vi "Log.StorePaths.vi"(8 "error in (no error)":errorcluster, 10 "TestStand Version (2013)":string, 11 "VeriStand Version (2013 SP1)":string) -> (0 "error out":errorcluster)   [LabVIEW 2013]
uses:
  <vilib>/Utility/sysdir.llb/System Directory Type.ctl
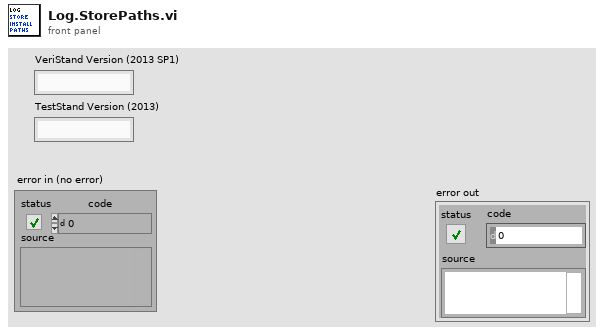
[diagram p1: front panel]
types:
  T1 = typedef "System Directory Type.ctl" = i32
  T2 = enum16{"open", "replace", "create", "open or create", "replace or create", "replace or create with confirmation"}
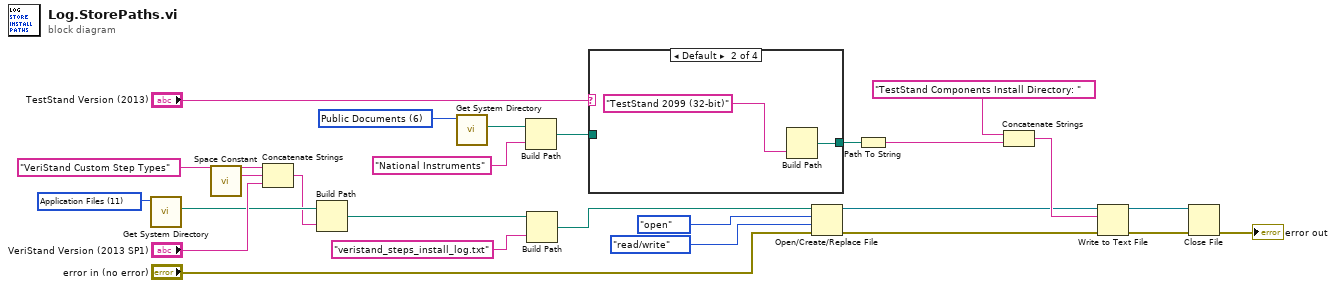
[diagram p0: block diagram]
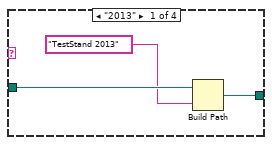
[diagram p2: hidden frame]
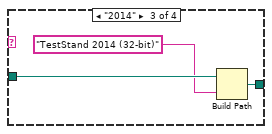
[diagram p3: hidden frame]
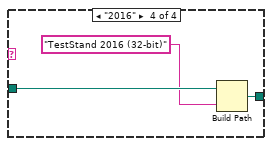
[diagram p4: hidden frame]
diagram:
  w18 = T1 6 items=["User Home"=0, "User Desktop"=1, "User Documents"=2, "User Application Data"=3, "User Preferences"=4, "User Temporary"=5, "Public Documents"=6, "Public Application Data"=7, "Public Preferences"=8, "Public Cache"=13, "System Core Libraries"=9, "System Installed Libraries"=10, "Application Files"=11, "Boot Volume Root"=12] ("system directory type")
  w25 = T1 11 items=["User Home"=0, "User Desktop"=1, "User Documents"=2, "User Application Data"=3, "User Preferences"=4, "User Temporary"=5, "Public Documents"=6, "Public Application Data"=7, "Public Preferences"=8, "Public Cache"=13, "System Core Libraries"=9, "System Installed Libraries"=10, "Application Files"=11, "Boot Volume Root"=12] ("system directory type")
  n1 = call <vilib>:"Get System Directory.vi"("system directory type"=w25) -> ("system directory"=w24:path)  [unwired: 10 in]
  n2 = call <vilib>:"Space Constant.vi"() -> ("String"=w22:string)
  n3 = Concatenate Strings("VeriStand Custom Step Types", w22, "VeriStand Version (2013 SP1)") -> (w21:string)
  n4 = Build Path(base path=w24, name or relative path=w21) -> (appended path=w3:path)
  n5 = call <vilib>:"Get System Directory.vi"("system directory type"=w18) -> ("system directory"=w17:path)  [unwired: 10 in]
  n6 = Build Path(base path=w17, name or relative path="National Instruments") -> (appended path=w14:path)
  n7 = Build Path(base path=w3, name or relative path="veristand_steps_install_log.txt") -> (appended path=w1:path)
  n8 = case shown="Default" "TestStand Version (2013)" {
    tunnel: w14 -> [w29 _ w34 w37]
    tunnel: [w27 w30 w32 w35] -> w13
    frame "2013" {
      n9 = Build Path(base path=w29, name or relative path="TestStand 2013") -> (appended path=w27:path)
    }
    frame Default {
      n10 = Build Path(name or relative path="TestStand 2099 (32-bit)") -> (appended path=w30:path)  [unwired: 1 in]
    }
    frame "2014" {
      n11 = Build Path(base path=w34, name or relative path="TestStand 2014 (32-bit)") -> (appended path=w32:path)
    }
    frame "2016" {
      n12 = Build Path(base path=w37, name or relative path="TestStand 2016 (32-bit)") -> (appended path=w35:path)
    }
  }
  n13 = Open/Create/Replace File(file path (use dialog)=w1, error in="error in (no error)", operation (0:open)=T2."open", access (0:read/write)=enum16{"read/write", "read-only", "write-only"}."read/write") -> (refnum out=w9:refnum<file>, error out=w8:errorcluster)  [unwired: 2 in, 1 out]
  n14 = Path To String(path=w13) -> (string=w11:string)
  n15 = Concatenate Strings("TestStand Components Install Directory: " ("name or relative path"), w11) -> (w10:string)
  n16 = Write to Text File(file (use dialog)=w9, text=w10, error in=w8) -> (refnum out=w6:refnum<file>, error out=w7:errorcluster)  [unwired: 1 in, 1 out]
  n17 = Close File(refnum=w6, error in=w7) -> (error out=→"error out":errorcluster)  [unwired: 1 out]
